vi "niRFUtil MASMT Util Resample_Create Prototype Filter (DBL).vi"(8 "error in (no error)":errorcluster, 10 "anti-aliasing?":bool=TRUE, 11 "FIR filter specifications":T1={"alias rejection (dB)"=120.0, "normalized bandwidth"=0.4536}) -> (0 "error out":errorcluster, 2 "decimation factor":i32, 3 "Coefficients":dbl[](array[numeric]))   [LabVIEW 2015, in "niRFUtil.lvlib"]
uses:
  niRFUtil.lvlib
  <vilib>/Analysis/NI_AALPro.lvlib
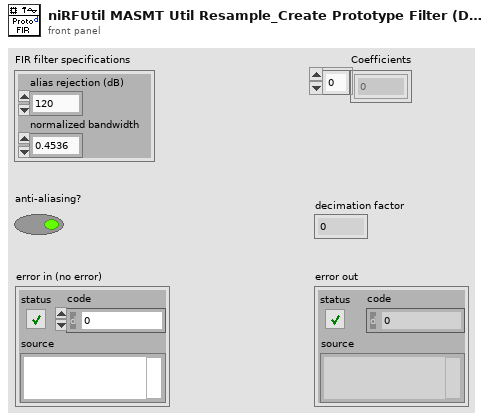
[diagram p1: front panel]
types:
  T1 = cluster{"alias rejection (dB)":dbl, "normalized bandwidth":dbl}
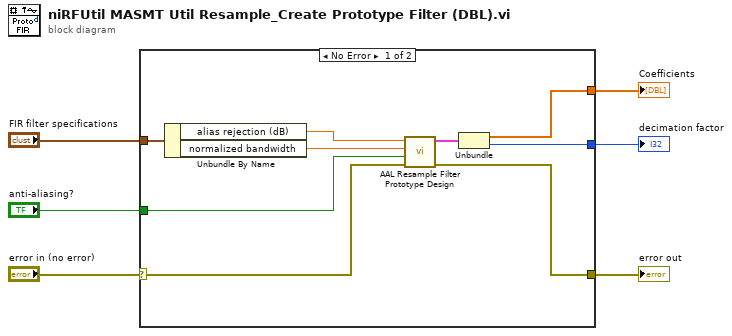
[diagram p0: block diagram]
diagram:
  n1 = case shown="No Error" "error in (no error)" {
    selector: "error in (no error)" -> [w10 w16]
    tunnel: [w14 _] -> w6
    tunnel: [w13 _] -> w5
    tunnel: "anti-aliasing?" -> [w12 _]
    tunnel: [w11 w16] -> w3
    tunnel: "FIR filter specifications" -> [w7 _]
    frame No Error {
      n2 = Unbundle By Name(w7) -> ("alias rejection (dB)"=w9:dbl, "normalized bandwidth"=w8:dbl)
      n3 = call <vilib>:"AAL Resample Filter Prototype Design.vi"("error in (no error)"=w10, "alias free"=w12, "normalized bandwidth"=w8, "A stop [dB]"=w9) -> ("error out"=w11:errorcluster, "filter prototype"=w15:cluster{"coefficients":dbl[], "factor":i32})  [unwired: 5 in, 1 out]
      n4 = Unbundle(w15) -> ("coefficients"=w14:dbl[], "factor"=w13:i32)
    }
    frame Error {
    }
  }
  "decimation factor" <- w5
  "Coefficients" <- w6
  "error out" <- w3
